vi "Tray_TrayTransformBool.vi"(8 "BOOLIN":bool[][](array[boolean])=[[FALSE, FALSE, FALSE, FALSE, FALSE, FALSE, FALSE], [FALSE, FALSE, TRUE, FALSE, FALSE, FALSE, FALSE], [FALSE, FALSE, FALSE, FALSE, FALSE, FALSE, FALSE], [FALSE, FALSE, FALSE, FALSE, FALSE, FALSE, FALSE], [FALSE, FALSE, FALSE, FALSE, FALSE, FALSE, FALSE], [FALSE, FALSE, FALSE, FALSE, FALSE, FALSE, FALSE], [FALSE, FALSE, FALSE, FALSE, FALSE, FALSE, FALSE], [FALSE, FALSE, FALSE, FALSE, FALSE, FALSE, FALSE], [FALSE, FALSE, FALSE, FALSE, FALSE, FALSE, FALSE]], 9 "StartNumber":i32, 10 "Direction":u16, 11 "TrayIn":cluster{"X":i32, "Y":i32}[][](array[cluster])) -> (2 "BoolOut":bool[][](array[boolean]), 3 "ArrayIndex":cluster{"X":i32, "Y":i32})   [LabVIEW 2014]
doc: "Direction\n\n0:L->R->U->D\n1:R->L->U->D\n2:L->R->D->U\n3:R->L->D->U\n4:U->D->L->R\n5:U->D->R->L\n6:D->U->L->R\n7:D->U->R->L"
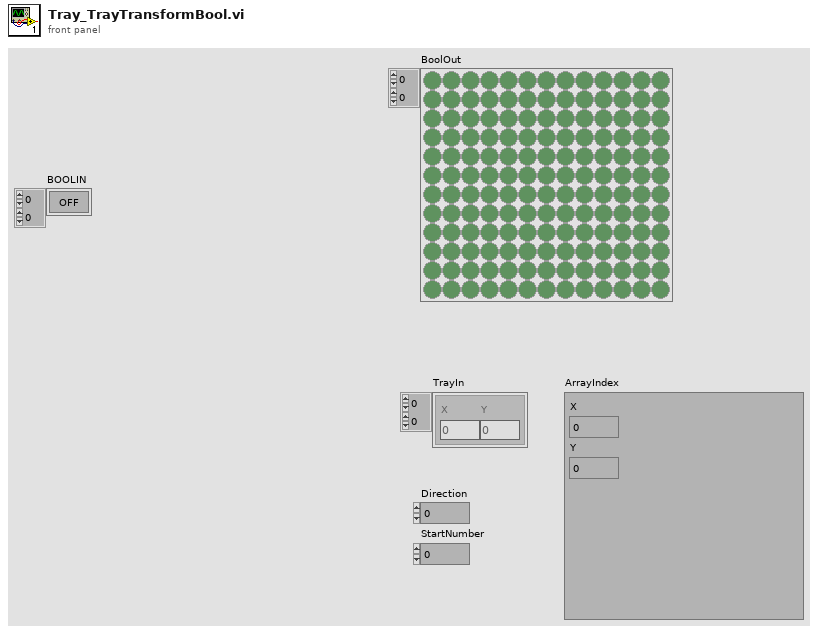
[diagram p1: front panel]
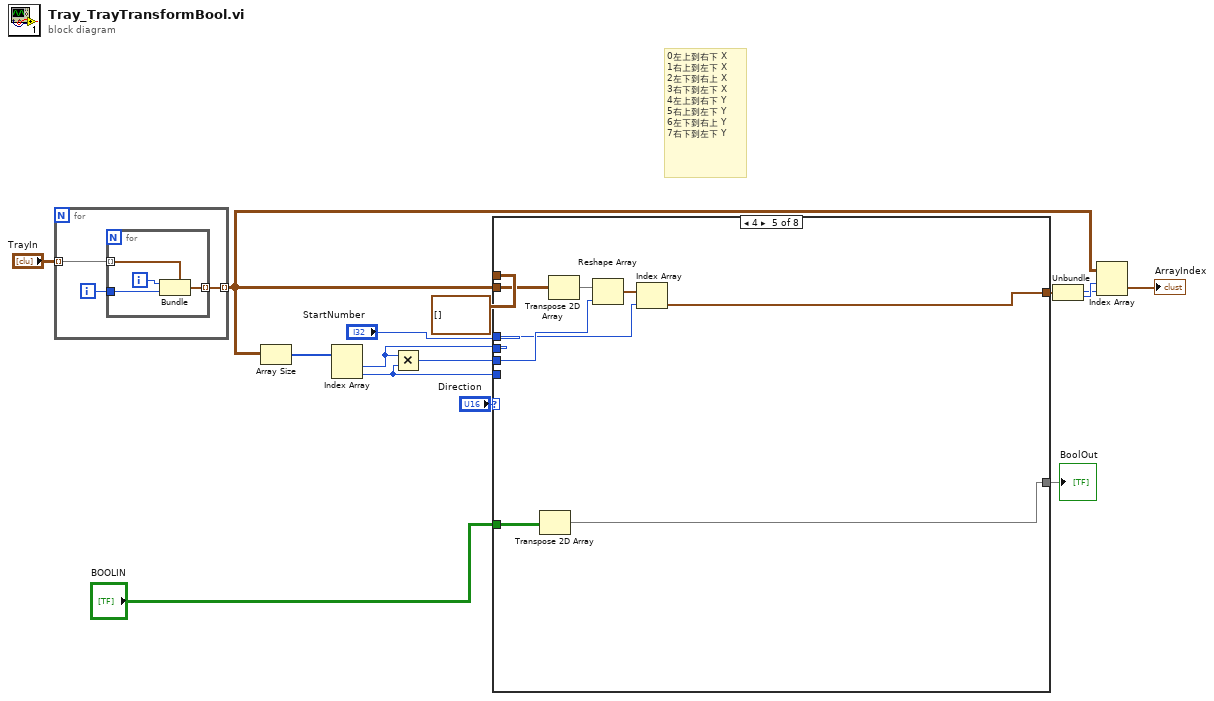
[diagram p0: block diagram]
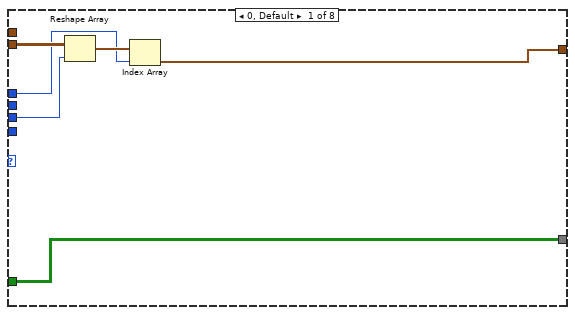
[diagram p2: hidden frame]
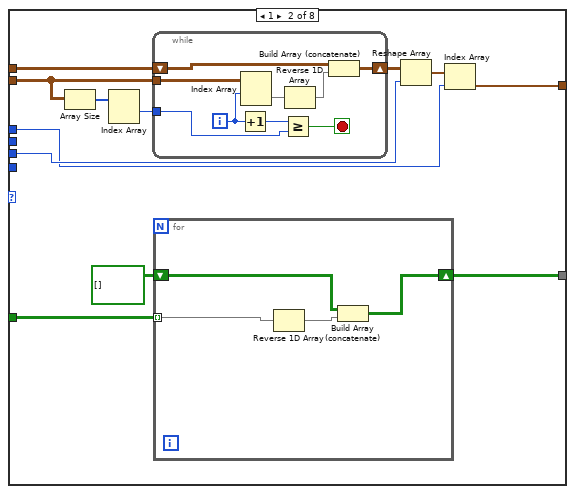
[diagram p3: hidden frame]
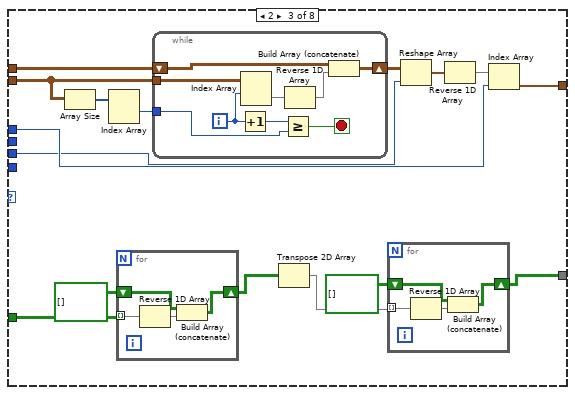
[diagram p4: hidden frame]
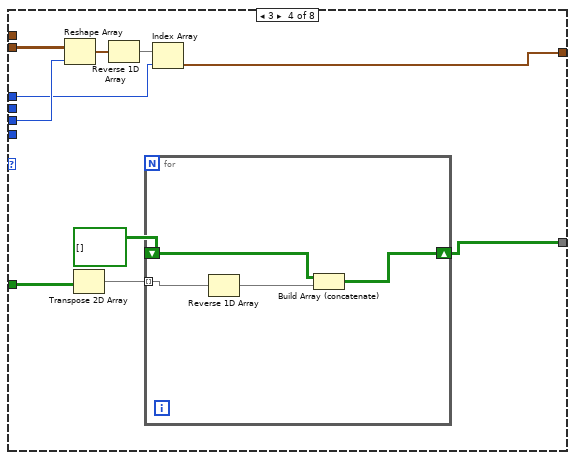
[diagram p5: hidden frame]
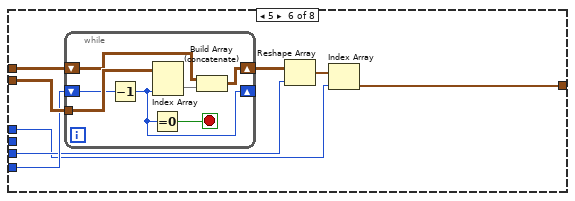
[diagram p6: hidden frame]
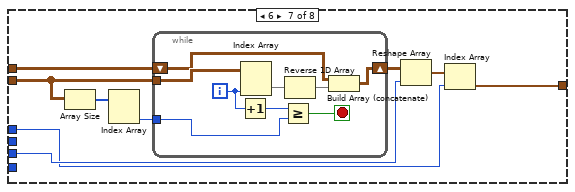
[diagram p7: hidden frame]
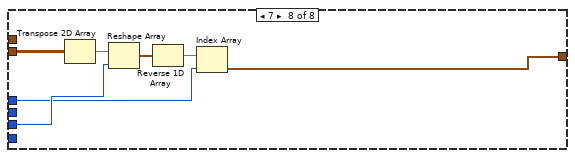
[diagram p8: hidden frame]
diagram:
  # "0左上到右下 X\n1右上到左下 X\n2左下到右上 X\n3右下到左下 X\n4左上到右下 Y\n5右上到左下 Y\n6左下到右上 Y\n7右下到左下 Y"
  n1 = for {
    tunnel: "TrayIn" -> [w18] mode=indexing
    tunnel: [w16] -> w10 mode=indexing
    i -> [w17]
    n2 = for {
      tunnel: w18 -> [w22] mode=indexing
      tunnel: w17 -> [w20]
      tunnel: [w19] -> w16 mode=indexing
      i -> [w21]
      n3 = Bundle(cluster=w22, "X"=w21, "Y"=w20) -> (w19:cluster{"X":i32, "Y":i32})
    }
  }
  n4 = Array Size(array=w10) -> (size(s)=w11:i32[])
  n5 = Index Array(array=w11) -> (element #1=w14:i32, element #2=w15:i32)  [unwired: 2 in]
  n6 = Multiply(x=w14, y=w15) -> (x*y=w13:i32)
  n7 = case shown="4" "Direction" {
    tunnel: "StartNumber" -> [w25 w32 w64 w91 w105 w113 w129 w145]
    tunnel: w10 -> [w28 w39 w65 w96 w108 w116 w131 w147]
    tunnel: w13 -> [w26 w33 w60 w92 w107 w114 w130 w146]
    tunnel: w14 -> [_ _ _ _ _ _ _ _]
    tunnel: w15 -> [_ _ _ _ _ w115 _ _]
    tunnel: [w24 w35 w62 w93 w103 w110 w125 w142] -> w9
    tunnel: cluster{"X":i32, "Y":i32}[][] [] ("TrayIn") -> [_ w34 w61 _ _ w109 w124 _]
    tunnel: "BOOLIN" -> [w23 w31 w57 w90 w102 _ _ _]
    tunnel: [w23 w29 w54 w87 w101 _ _ _] -> w1
    frame 0, Default {
      n8 = Reshape Array(w28, w26) -> (w27:cluster{"X":i32, "Y":i32}[])
      n9 = Index Array(array=w27, index=w25) -> (element=w24:cluster{"X":i32, "Y":i32})
    }
    frame 1 {
      n10 = Array Size(array=w39) -> (size(s)=w40:i32[])
      n11 = Index Array(array=w40) -> (element #1=w37:i32)  [unwired: 2 in, 1 out]
      n12 = while {
        tunnel: w39 -> [w53]
        shift-right: [w48] -> w38
        shift-left: w34 -> [w49]
        tunnel: w37 -> [w45]
        i -> [w51]
        stop <- w52 stop-if-true
        n13 = Increment(x=w51) -> (x+1=w46:i32)
        n14 = Index Array(array=w53, index (row)=w51) -> (element=w50:cluster{"X":i32, "Y":i32}[])  [unwired: 1 in]
        n15 = Greater Or Equal?(x=w46, y=w45) -> (x >= y?=w52:bool)
        n16 = Reverse 1D Array(array=w50) -> (reversed array=w47:cluster{"X":i32, "Y":i32}[])
        n17 = Build Array (concatenate)(w49, w47) -> (w48:cluster{"X":i32, "Y":i32}[][])
      }
      n18 = for {
        tunnel: w31 -> [w44] mode=indexing
        shift-right: [w42] -> w29
        shift-left: bool[][] [] -> [w41]
        n19 = Reverse 1D Array(array=w44) -> (reversed array=w43:bool[])
        n20 = Build Array (concatenate)(w41, w43) -> (w42:bool[][])
      }
      n21 = Reshape Array(w38, w33) -> (w36:cluster{"X":i32, "Y":i32}[])
      n22 = Index Array(array=w36, index=w32) -> (element=w35:cluster{"X":i32, "Y":i32})
    }
    frame 2 {
      n23 = Array Size(array=w65) -> (size(s)=w69:i32[])
      n24 = Index Array(array=w69) -> (element #1=w66:i32)  [unwired: 2 in, 1 out]
      n25 = for {
        tunnel: w57 -> [w77] mode=indexing
        shift-right: [w75] -> w58
        shift-left: bool[][] [] -> [w74]
        n26 = Reverse 1D Array(array=w77) -> (reversed array=w76:bool[])
        n27 = Build Array (concatenate)(w74, w76) -> (w75:bool[][])
      }
      n28 = while {
        tunnel: w65 -> [w86]
        shift-right: [w81] -> w68
        shift-left: w61 -> [w82]
        tunnel: w66 -> [w78]
        i -> [w84]
        stop <- w85 stop-if-true
        n29 = Increment(x=w84) -> (x+1=w79:i32)
        n30 = Index Array(array=w86, index (row)=w84) -> (element=w83:cluster{"X":i32, "Y":i32}[])  [unwired: 1 in]
        n31 = Greater Or Equal?(x=w79, y=w78) -> (x >= y?=w85:bool)
        n32 = Reverse 1D Array(array=w83) -> (reversed array=w80:cluster{"X":i32, "Y":i32}[])
        n33 = Build Array (concatenate)(w82, w80) -> (w81:cluster{"X":i32, "Y":i32}[][])
      }
      n34 = Transpose 2D Array(2D array=w58) -> (transposed array=w55:bool[][])
      n35 = for {
        tunnel: w55 -> [w73] mode=indexing
        shift-right: [w71] -> w54
        shift-left: bool[][] [] -> [w70]
        n36 = Reverse 1D Array(array=w73) -> (reversed array=w72:bool[])
        n37 = Build Array (concatenate)(w70, w72) -> (w71:bool[][])
      }
      n38 = Reshape Array(w68, w60) -> (w67:cluster{"X":i32, "Y":i32}[])
      n39 = Reverse 1D Array(array=w67) -> (reversed array=w63:cluster{"X":i32, "Y":i32}[])
      n40 = Index Array(array=w63, index=w64) -> (element=w62:cluster{"X":i32, "Y":i32})
    }
    frame 3 {
      n41 = Reshape Array(w96, w92) -> (w95:cluster{"X":i32, "Y":i32}[])
      n42 = Transpose 2D Array(2D array=w90) -> (transposed array=w89:bool[][])
      n43 = Reverse 1D Array(array=w95) -> (reversed array=w94:cluster{"X":i32, "Y":i32}[])
      n44 = for {
        tunnel: w89 -> [w100] mode=indexing
        shift-right: [w98] -> w87
        shift-left: bool[][] [] -> [w97]
        n45 = Reverse 1D Array(array=w100) -> (reversed array=w99:bool[])
        n46 = Build Array (concatenate)(w97, w99) -> (w98:bool[][])
      }
      n47 = Index Array(array=w94, index=w91) -> (element=w93:cluster{"X":i32, "Y":i32})
    }
    frame 4 {
      n48 = Transpose 2D Array(2D array=w102) -> (transposed array=w101:bool[][])
      n49 = Transpose 2D Array(2D array=w108) -> (transposed array=w104:cluster{"X":i32, "Y":i32}[][])
      n50 = Reshape Array(w104, w107) -> (w106:cluster{"X":i32, "Y":i32}[])
      n51 = Index Array(array=w106, index=w105) -> (element=w103:cluster{"X":i32, "Y":i32})
    }
    frame 5 {
      n52 = while {
        tunnel: w116 -> [w123]
        shift-right: [w120] -> w112
        shift-left: w109 -> [w121]
        shift-right: [w118] -> _
        shift-left: w115 -> [w119]
        stop <- w122 stop-if-true
        n53 = Decrement(x=w119) -> (x-1=w118:i32)
        n54 = Equal To 0?(x=w118) -> (x = 0?=w122:bool)
        n55 = Index Array(array=w123, index (col)=w118) -> (element=w117:cluster{"X":i32, "Y":i32}[])  [unwired: 1 in]
        n56 = Build Array (concatenate)(w121, w117) -> (w120:cluster{"X":i32, "Y":i32}[][])
      }
      n57 = Reshape Array(w112, w114) -> (w111:cluster{"X":i32, "Y":i32}[])
      n58 = Index Array(array=w111, index=w113) -> (element=w110:cluster{"X":i32, "Y":i32})
    }
    frame 6 {
      n59 = Array Size(array=w131) -> (size(s)=w132:i32[])
      n60 = Index Array(array=w132) -> (element #2=w128:i32)  [unwired: 2 in, 1 out]
      n61 = while {
        tunnel: w131 -> [w141]
        shift-right: [w137] -> w126
        shift-left: w124 -> [w138]
        tunnel: w128 -> [w134]
        i -> [w133]
        stop <- w140 stop-if-true
        n62 = Increment(x=w133) -> (x+1=w135:i32)
        n63 = Index Array(array=w141, index (col)=w133) -> (element=w139:cluster{"X":i32, "Y":i32}[])  [unwired: 1 in]
        n64 = Greater Or Equal?(x=w135, y=w134) -> (x >= y?=w140:bool)
        n65 = Reverse 1D Array(array=w139) -> (reversed array=w136:cluster{"X":i32, "Y":i32}[])
        n66 = Build Array (concatenate)(w138, w136) -> (w137:cluster{"X":i32, "Y":i32}[][])
      }
      n67 = Reshape Array(w126, w130) -> (w127:cluster{"X":i32, "Y":i32}[])
      n68 = Index Array(array=w127, index=w129) -> (element=w125:cluster{"X":i32, "Y":i32})
    }
    frame 7 {
      n69 = Transpose 2D Array(2D array=w147) -> (transposed array=w144:cluster{"X":i32, "Y":i32}[][])
      n70 = Reshape Array(w144, w146) -> (w148:cluster{"X":i32, "Y":i32}[])
      n71 = Reverse 1D Array(array=w148) -> (reversed array=w143:cluster{"X":i32, "Y":i32}[])
      n72 = Index Array(array=w143, index=w145) -> (element=w142:cluster{"X":i32, "Y":i32})
    }
  }
  "BoolOut" <- w1
  n73 = Unbundle(w9) -> ("X"=w4:i32, "Y"=w5:i32)
  n74 = Index Array(array=w10, index (row)=w5, index (col)=w4) -> (element=→"ArrayIndex":cluster{"X":i32, "Y":i32})
